vi "Handle setAllData.vi"(8 "error in (no error)":errorcluster, 10 "AllData":variant, 11 "instrument.PPMS in":refnum<class "instrument.PPMS.lvclass">) -> (0 "error out":errorcluster, 3 "instrument.PPMS out":refnum<class "instrument.PPMS.lvclass">)   [LabVIEW 2019, in "instrument.PPMS.lvclass"]
doc: "Override to handle \"getAll\" or \"getAllData\" commands for <b>your</b> Instrument"
uses:
  instrument.PPMS.lvclass
  Typedefs/PPMS.getAll--cluster.ctl
  instrument.PPMS.lvclass/instrument.PPMS.ctl
  b6f22601-2e15-4185-a506-94e6a3522059.vi
  <vilib>/JDP Science/JSONtext/JSON text to Variant.vi
  <vilib>/JDP Science/JSONtext/LVClass Serializer/JSONtext LVClass Serializer.lvclass
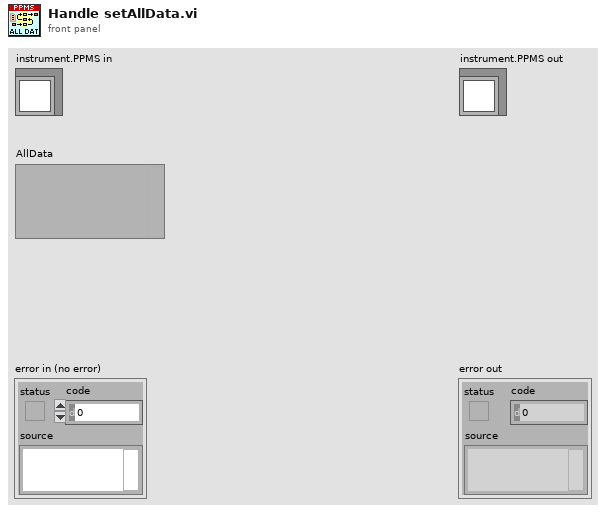
[diagram p1: front panel]
types:
  T1 = typedef "instrument.PPMS.lvclass/PPMS.getAll--cluster.ctl" = cluster{"Chamber Status":string, "Helium Level":dbl, "Temperature":dbl, "Temperature Status":string, "Magnetic Field":dbl, "Magnet Status":string, "Position":dbl}
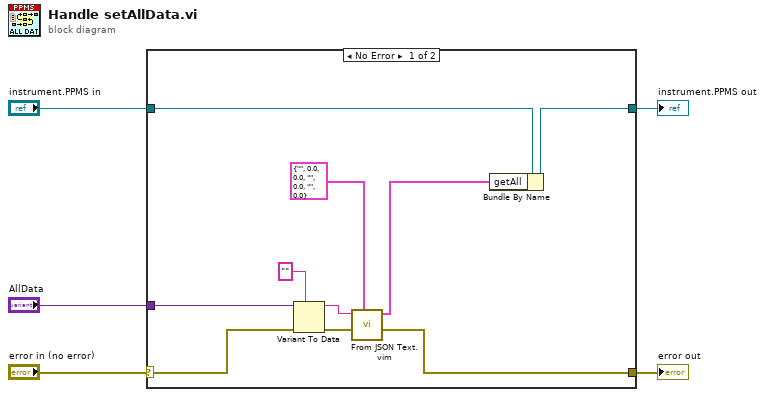
[diagram p0: block diagram]
diagram:
  n1 = case shown="No Error" "error in (no error)" {
    selector: "error in (no error)" -> [w11 w17]
    tunnel: [w10 w17] -> w2
    tunnel: [w8 w16] -> w5
    tunnel: "instrument.PPMS in" -> [w7 w16]
    tunnel: "AllData" -> [w6 _]
    frame No Error {
      n2 = Variant To Data(error in=w11, type="", Variant=w6) -> (data=w14:string, error out=w13:errorcluster)
      n3 = call "From JSON Text.vim"("Data Type and Default Value"=T1 {"Chamber Status"="", "Helium Level"=0.0, "Temperature"=0.0, "Temperature Status"="", "Magnetic Field"=0.0, "Magnet Status"="", "Position"=0.0} ("getAll"), "error in (no error)"=w13, "JSON"=w14) -> ("error out"=w10:errorcluster, "Data out"=w9:T1)  [unwired: 7 in]
      n4 = Bundle By Name(cluster=w7, "getAll"=w9) -> (w8:refnum<class "instrument.PPMS.lvclass">)
    }
    frame Error {
    }
  }
  "error out" <- w2
  "instrument.PPMS out" <- w5
